vi "mysqlDbConnectivity.vi"() -> ()   [LabVIEW 2025]
uses:
  <vilib>/addons/database/Connection.llb/DB Tools Open Connec (String).vi
  <vilib>/addons/database/Connection.llb/Conn Execute.vi
  <vilib>/addons/database/Recordset.llb/Rec Fetch Recordset Data (R).vi
  <vilib>/addons/database/_DB Variant To Data/Database Variant To Data.xnode
  <vilib>/addons/database/NI_Database_API.lvlib
panel:
  in  "Multicolumn Listbox":i32(listbox)
  out "Array 3":string[][](array[string])
  out "Array 2":string[][](array[string])
  out "Array":string[][](array[string])
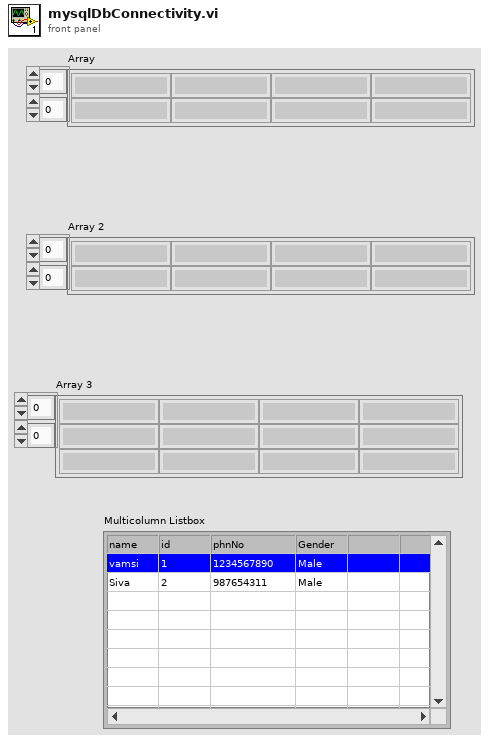
[diagram p1: front panel]
types:
  T1 = typedef "NI_Database_API.lvlib/Conn ObjectReference.ctl" = refnum<k1>
  T2 = typedef "NI_Database_API.lvlib/Rec ObjectReference.ctl" = refnum<k1>
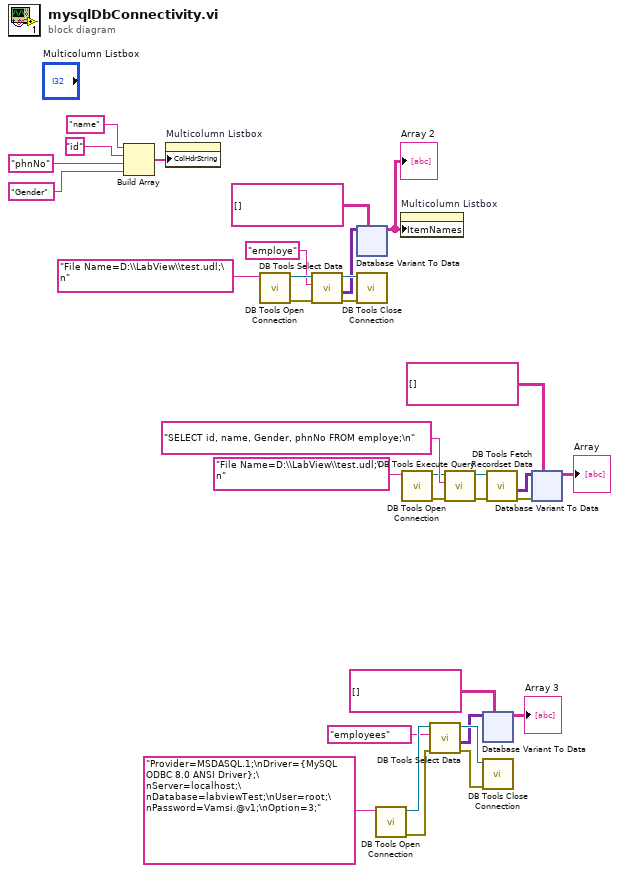
[diagram p0: block diagram]
diagram:
  n1 = Build Array("name", "id", "phnNo", "Gender") -> (w1:string[])
  n2 = property on="Multicolumn Listbox" class="MCListbox (strict)"("ColHdrString"=w1) -> ()  [unwired: 2 in, 2 out]
  n3 = call-poly <vilib>:"DB Tools Open Connection.vi"("connection information"="File Name=D:\\LabView\\test.udl;\n") -> ("error out"=w22:errorcluster, "connection reference"=w21:T1)  [unwired: 7 in]
  n4 = call <vilib>:"DB Tools Select Data.vi"("error in (no error)"=w22, "table"="employe", "connection reference"=w21) -> ("error out"=w19:errorcluster, "data"=w17:variant[][], "connection reference out"=w20:T1)  [unwired: 3 in]
  n5 = xnode "Database Variant To Data"("database variant"=w17, "type"=string[][] []) -> ("data"=w6:string[][])  [unwired: 1 in, 1 out]
  "Array 2" <- w6
  n6 = call <vilib>:"DB Tools Close Connection.vi"("error in (no error)"=w19, "connection reference"=w20) -> ()  [unwired: 5 in, 1 out]
  n7 = call-poly <vilib>:"DB Tools Open Connection.vi"("connection information"="Provider=MSDASQL.1;\nDriver={MySQL ODBC 8.0 ANSI Driver};\nServer=localhost;\nDatabase=labviewTest;\nUser=root;\nPassword=Vamsi.@v1;\nOption=3;") -> ("error out"=w14:errorcluster, "connection reference"=w15:T1)  [unwired: 7 in]
  n8 = property on="Multicolumn Listbox" class="MCListbox (strict)"("ItemNames"=w6) -> ()  [unwired: 2 in, 2 out]
  n9 = call-poly <vilib>:"DB Tools Open Connection.vi"("connection information"="File Name=D:\\LabView\\test.udl;\n") -> ("error out"=w24:errorcluster, "connection reference"=w25:T1)  [unwired: 7 in]
  n10 = call <vilib>:"DB Tools Select Data.vi"("error in (no error)"=w14, "table"="employees", "connection reference"=w15) -> ("error out"=w12:errorcluster, "data"=w7:variant[][], "connection reference out"=w13:T1)  [unwired: 3 in]
  n11 = call-poly <vilib>:"DB Tools Execute Query.vi"("error in (no error)"=w24, "SQL query"="SELECT id, name, Gender, phnNo FROM employe;\n", "connection reference"=w25) -> ("error out"=w32:errorcluster, "recordset reference"=w29:T2)  [unwired: 5 in]
  n12 = xnode "Database Variant To Data"("database variant"=w7, "type"=string[][] []) -> ("data"=→"Array 3":string[][])  [unwired: 1 in, 1 out]
  n13 = call <vilib>:"DB Tools Close Connection.vi"("error in (no error)"=w12, "connection reference"=w13) -> ()  [unwired: 5 in, 1 out]
  n14 = call-poly <vilib>:"DB Tools Fetch Recordset Data.vi"("error in (no error)"=w32, "recordset reference"=w29) -> ("error out"=w31:errorcluster, "recordset data"=w28:variant[][])  [unwired: 3 in, 1 out]
  n15 = xnode "Database Variant To Data"("database variant"=w28, "error in (no error)"=w31, "type"=string[][] []) -> ("data"=→"Array":string[][])  [unwired: 1 out]
